vi "Read Filter array temp.vi"(8 "error in (no error)":errorcluster, 11 "Filter params in":refnum<class "CV-Filter.lvclass">) -> (0 "error out":errorcluster, 2 "Filter array temp":T1[](array[typedef]), 3 "Filter params out":refnum<class "CV-Filter.lvclass">)   [LabVIEW 2013, in "CameraVision.lvlib" / "CV-Filter.lvclass"]
uses:
  CV-Filter.lvclass
  Filter-settings.ctl
  Filter-characteristic.ctl
  CV-Filter.lvclass/CV-Filter.ctl
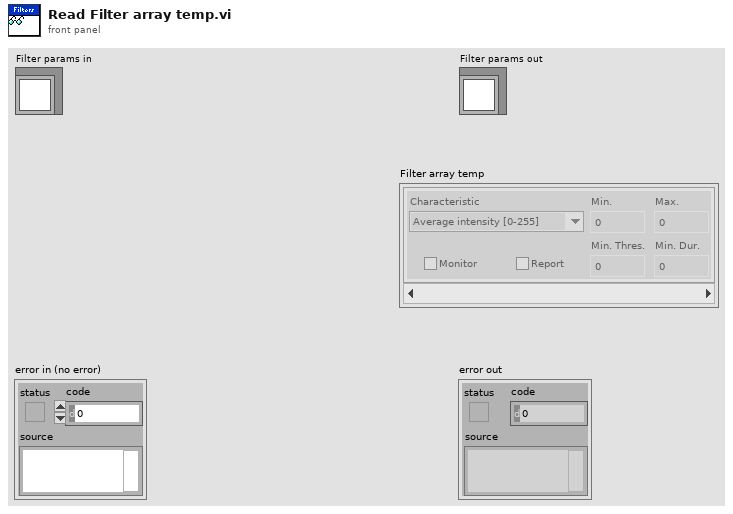
[diagram p1: front panel]
types:
  T1 = typedef "CameraVision.lvlib/CV-Filter.lvclass/Filter-settings.ctl" = cluster{"Characteristic":T2, "Monitor":bool, "Min.":dbl, "Max.":dbl, "Min. Thres.":dbl, "Min. Dur.":u16, "Report":bool}
  T2 = typedef "CameraVision.lvlib/CV-Filter.lvclass/Filter-characteristic.ctl" = enum16{"Average intensity [0-255]", "Peak intensity [0-255]", "Melt-pool size [mm²]", "Melt-pool aspect ratio []", "Melt-pool fragments []", "Melt-pool position X [pixel]", "Melt-pool position Y [pixel]", "Average temperature [°C]", "Max. temperature [°C]", "Min. temperature [°C]", "Std. dev. temperature [°C]"}
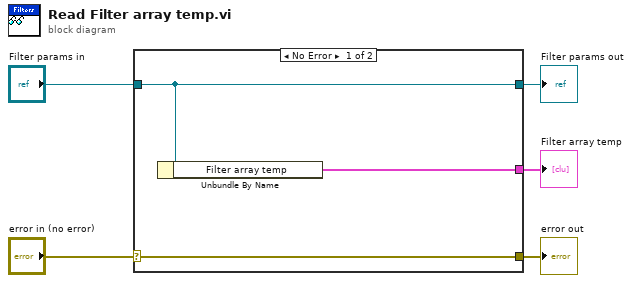
[diagram p0: block diagram]
diagram:
  n1 = case shown="No Error" "error in (no error)" {
    selector: "error in (no error)" -> [w8 w9]
    tunnel: [w8 w9] -> w4
    tunnel: [w7 w10] -> w2
    tunnel: "Filter params in" -> [w7 w10]
    tunnel: [w6 _] -> w1
    frame No Error {
      n2 = Unbundle By Name(w7) -> ("Filter array temp"=w6:T1[])
    }
    frame Error {
    }
  }
  "error out" <- w4
  "Filter params out" <- w2
  "Filter array temp" <- w1
